vi "Check_Module_Information.vi"(0 "Address Cluster":T1 {"tsl_communcation_method" items=["GPIB", "C232C", "TCPIP", "USB"]; "MPM_communcation_method" items=["GPIB", "C232C", "TCPIP", "USB"]}, 3 "错误输入（无错误）":errorcluster caption="error in") -> (7 "Address Cluster out":T1 {"tsl_communcation_method" items=["GPIB", "C232C", "TCPIP", "USB"]; "MPM_communcation_method" items=["GPIB", "C232C", "TCPIP", "USB"]}, 8 "Flag_215":bool, 9 "Flag_213":bool, 10 "error out":errorcluster)   [LabVIEW 2017]
doc: "check Module information inside system"
uses:
  CTL/Address Cluster.ctl
  D:/test/ILSTS/LV_IL_Sample/DLL/InstrumentDLL.dll
  DLL/InstrumentDLL.dll
panel:
  in  "counter_215":i32
  in  "enable_module_count":i32
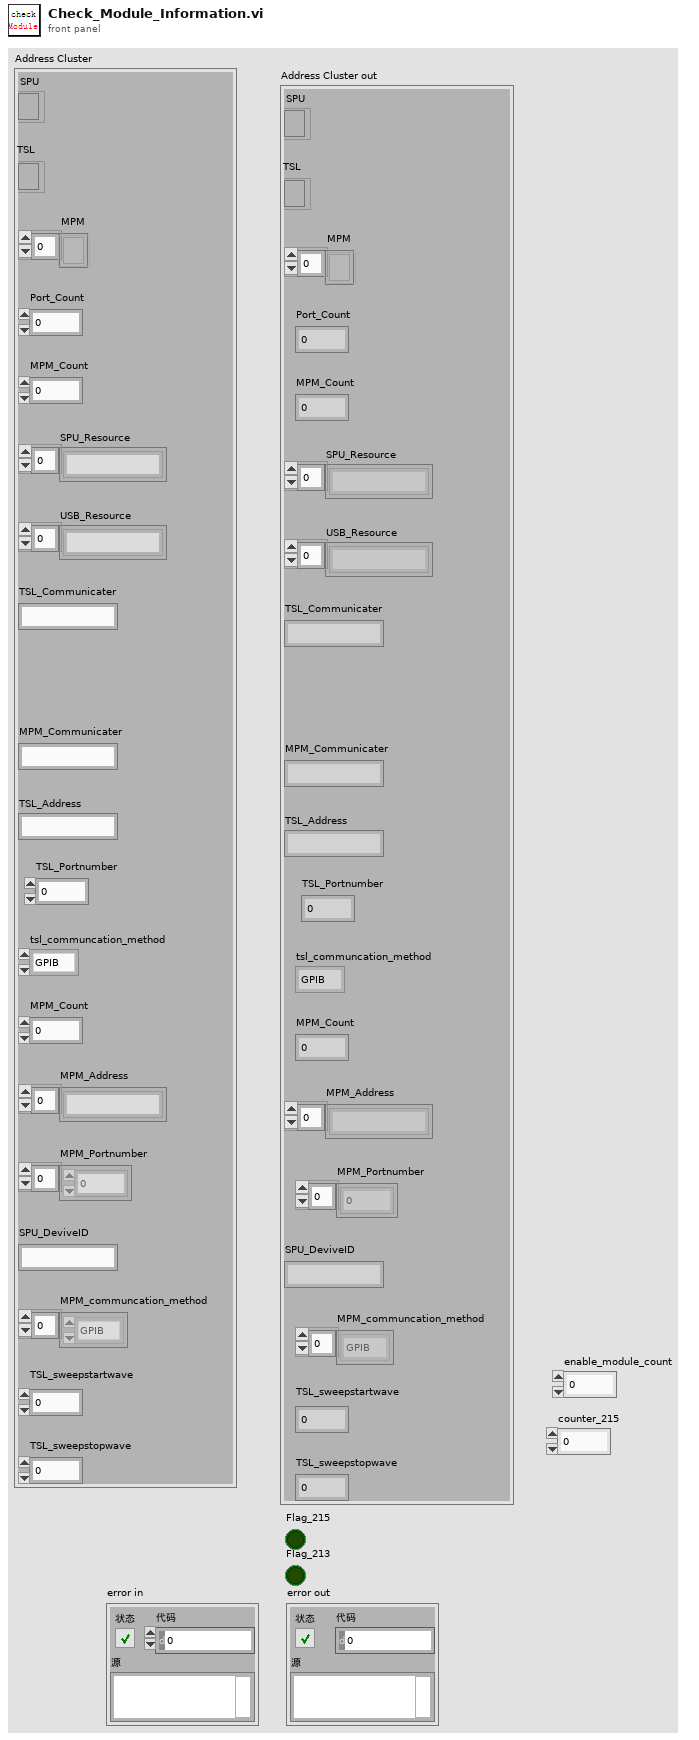
[diagram p1: front panel]
types:
  T1 = typedef "Address Cluster.ctl" = cluster{"SPU":refnum<k24>, "MPM":refnum<k24>[], "Port_Count":dbl, "MPM_Count":dbl, "SPU_Resource":string[], "USB_Resource":string[], "MPM_Communicater":string, "MPM_Count":dbl, "MPM_Address":string[], "MPM_Portnumber":dbl[], "SPU_DeviveID":string, "MPM_communcation_method":i32[], "TSL_sweepstartwave":dbl, "TSL_sweepstopwave":dbl, "TSL_Address":string, "TSL_Communicater":string, "TSL":refnum<k24>, "tsl_communcation_method":i32, "TSL_Portnumber":dbl}
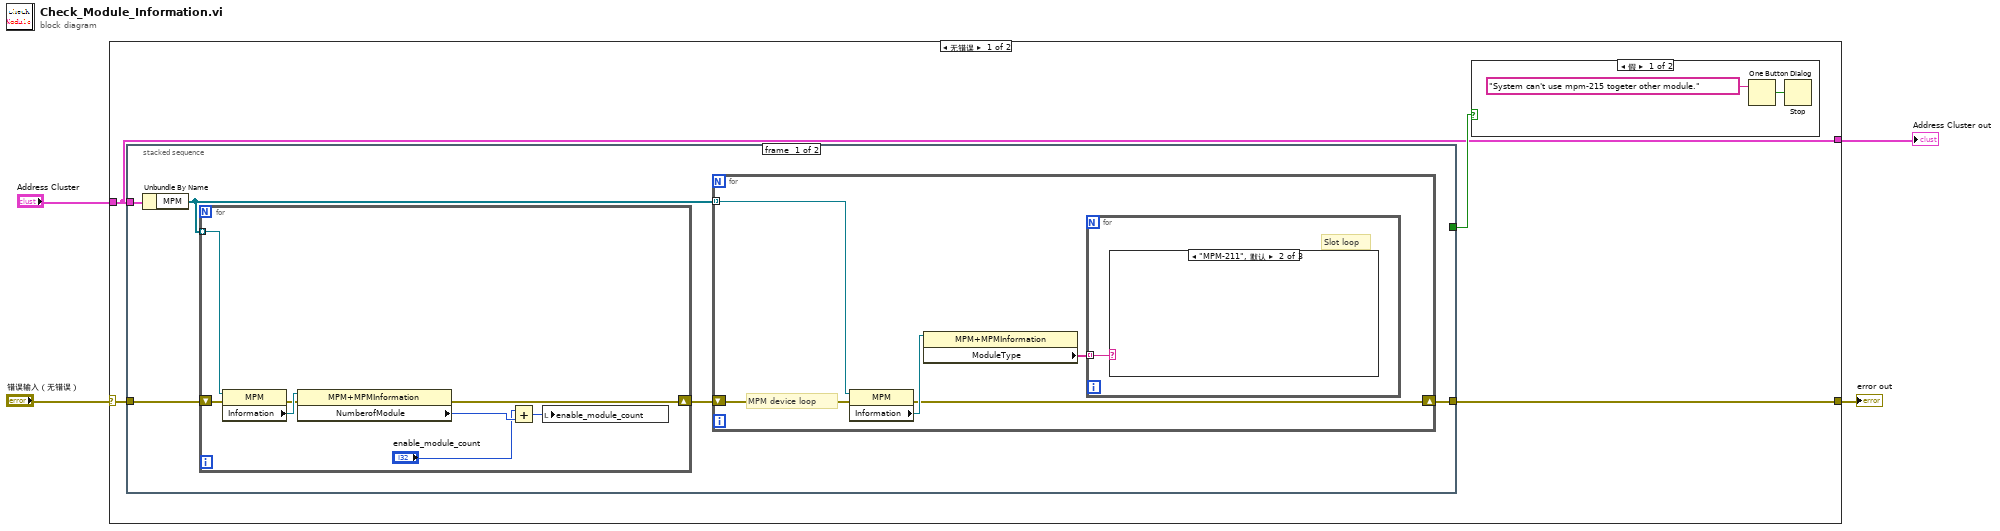
[diagram p0: block diagram]
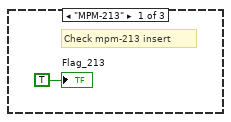
[diagram p3: hidden frame]
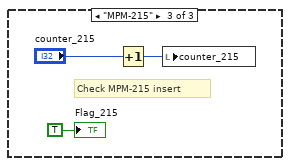
[diagram p4: hidden frame]
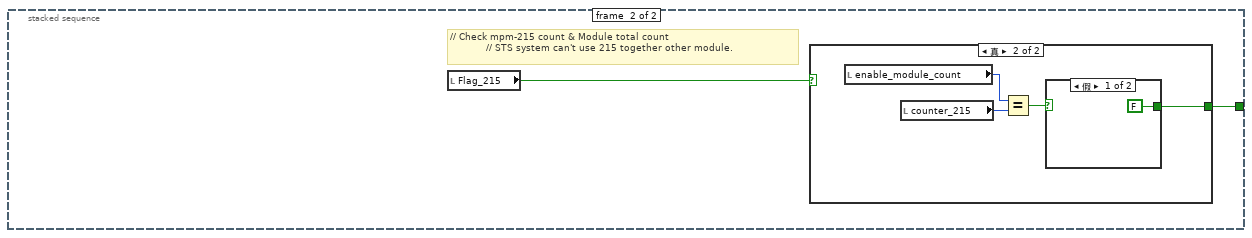
[diagram p5: hidden frame]
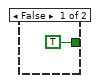
[diagram p6: hidden frame]
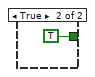
[diagram p7: hidden frame]
diagram:
  n1 = case shown="无错误" "错误输入（无错误）" {
    selector: "错误输入（无错误）" -> [w7 w44]
    tunnel: "Address Cluster" -> [w5 w43]
    tunnel: [w6 w44] -> w2
    tunnel: [w5 w43] -> w1
    frame No Error {
      n2 = stacked-sequence {
        tunnel: w5 -> [w15 _]
        tunnel: [_ w34] -> w8
        tunnel: w7 -> [w13 _]
        tunnel: [w11 _] -> w6
        frame #0 {
          n3 = Unbundle By Name(w15) -> ("MPM"=w14:refnum<k24>[])
          n4 = for {
            tunnel: w14 -> [w23] mode=indexing
            shift-right: [w16] -> w12
            shift-left: w13 -> [w18]
            n5 = property on="属性节点" class="MPM"(reference=w23, error in=w18) -> (error out=w17:errorcluster, "Information"=w22:refnum<k24>)  [unwired: 1 out]
            n6 = property class="MPM+MPMInformation"(reference=w22, error in=w17) -> (error out=w16:errorcluster, "NumberofModule"=w21:i32)  [unwired: 1 out]
            n7 = Add(x="enable_module_count", y=w21) -> (x+y=w19:i32)
            n8 = local write "enable_module_count"(w19) -> ()
          }
          n9 = for {
            tunnel: w14 -> [w28] mode=indexing
            shift-right: [w24] -> w11
            shift-left: w12 -> [w25]
            # "MPM device loop"
            n10 = property on="属性节点" class="MPM"(reference=w28, error in=w25) -> (error out=w24:errorcluster, "Information"=w27:refnum<k24>)  [unwired: 1 out]
            n11 = property class="MPM+MPMInformation"(reference=w27) -> ("ModuleType"=w26:string[])  [unwired: 1 in, 2 out]
            n12 = for {
              tunnel: w26 -> [w29] mode=indexing
              # "Slot loop"
              n13 = case shown="\"MPM-211\", 默认" w29 {
                frame "MPM-213" {
                  # "Check mpm-213 insert"
                  "Flag_213" <- TRUE ("Flag_213")
                }
                frame "MPM-211", Default {
                }
                frame "MPM-215" {
                  # "Check MPM-215 insert"
                  n14 = Increment(x="counter_215") -> (x+1=w31:i32)
                  n15 = local write "counter_215"(w31) -> ()
                  "Flag_215" <- TRUE ("Flag_215")
                }
              }
            }
          }
        }
        frame #1 {
          # "// Check mpm-215 count & Module total count\n            // STS system can't use 215 together other module."
          n16 = local read "Flag_215"() -> (w35:bool)
          n17 = case shown="真" w35 {
            tunnel: [TRUE w37] -> w34
            frame False {
            }
            frame True {
              n18 = local read "enable_module_count"() -> (w40:i32)
              n19 = local read "counter_215"() -> (w39:i32)
              n20 = Equal?(x=w40, y=w39) -> (x = y?=w38:bool)
              n21 = case shown="假" w38 {
                tunnel: [FALSE TRUE] -> w37
                frame False {
                }
                frame True {
                }
              }
            }
          }
        }
      }
      n22 = case shown="假" w8 {
        frame False {
          n23 = One Button Dialog(message="System can't use mpm-215 togeter other module." ("消息")) -> (true=w9:bool)  [unwired: 1 in]
          n24 = Stop(stop? (T)=w9) -> ()
        }
        frame True {
        }
      }
    }
    frame Error {
    }
  }
  "Address Cluster out" <- w1
  "error out" <- w2
